vi "AudioTest.SoundCheck Data Log Analysis_Module - Load Data Task.vi"(7 "Q Name":string="AudioGraphs", 8 "error in (no error)":errorcluster, 9 "UUT Folder":path) -> (0 "error out":errorcluster)   [LabVIEW 2018]
uses:
  <vilib>/KATE/Queues/Queue Utils.lvlib
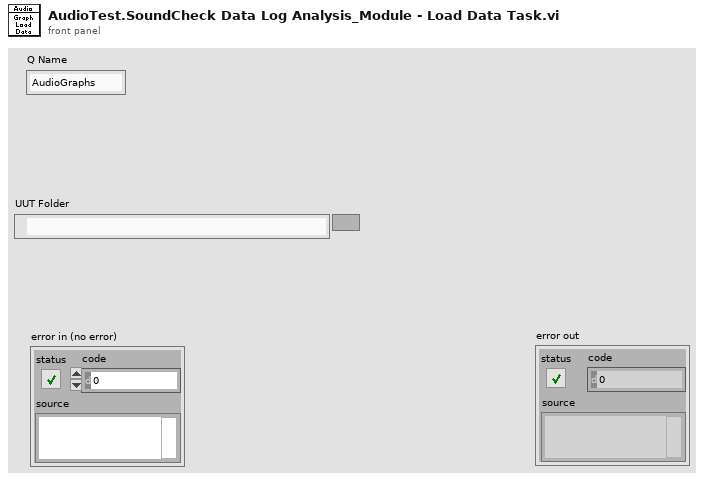
[diagram p1: front panel]
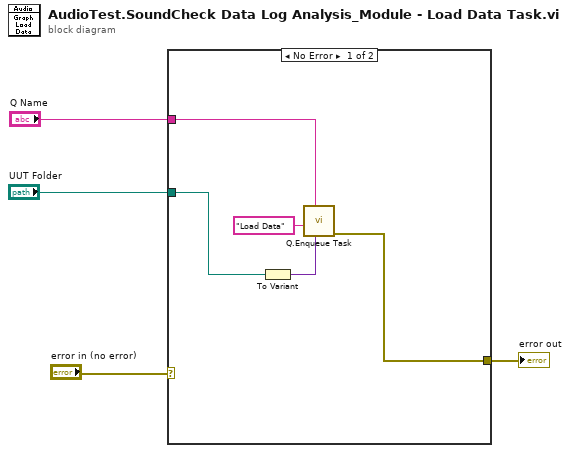
[diagram p0: block diagram]
diagram:
  n1 = case shown="No Error" "error in (no error)" {
    selector: "error in (no error)" -> [_ w10]
    tunnel: "Q Name" -> [w9 _]
    tunnel: "UUT Folder" -> [w7 _]
    tunnel: [w6 w10] -> w1
    frame No Error {
      n2 = To Variant(anything=w7) -> (Variant=w8:variant)
      n3 = call <vilib>:"Q.Enqueue Task.vi"("Data1"=w8, "Q Name"=w9, "Task Name"="Load Data") -> ("error out"=w6:errorcluster)  [unwired: 7 in, 1 out]
    }
    frame Error {
    }
  }
  "error out" <- w1
